vi "Update Z Cursors.vi"(8 "error in (no error)":errorcluster, 11 "Analysis Graph in":refnum<class "Analysis Graph.lvclass">) -> (0 "error out":errorcluster, 3 "Analysis Graph out":refnum<class "Analysis Graph.lvclass">)   [LabVIEW 2023, in "Analysis Graph.lvclass"]
uses:
  Analysis Graph.lvclass
  D:/git/Graph-Classes/source/Series Graph/Series Graph.lvclass
  Series Graph/Series Graph.lvclass/Series Graph.ctl
  Analysis Graph.lvclass/Analysis Graph.ctl
  Series Graph/Series Graph.lvclass
  D:/git/Graph-Classes/source/Detail Graph/Detail Graph.lvclass
  D:/git/Graph-Classes/source/Base Graph/Base Graph.lvclass
  D:/git/Graph-Classes/source/Analysis Graph/Analysis Graph.lvclass
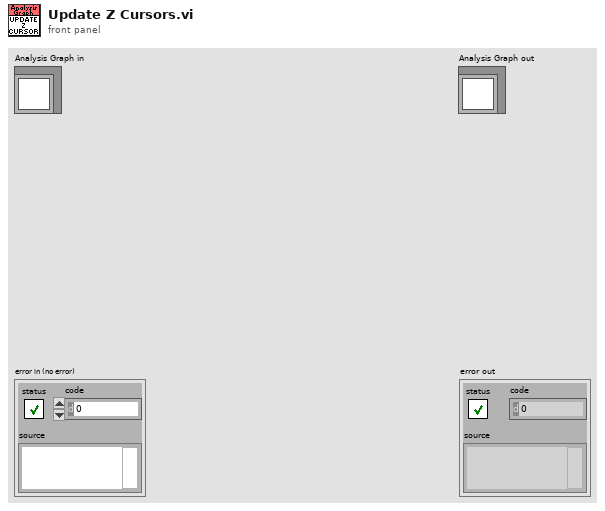
[diagram p1: front panel]
types:
  T1 = cluster{"ROI X":cluster{"Index":u32, "Length":u32}, "ROI Y":cluster{"Index":u32, "Length":u32}, "ROI Z":cluster{"Index":u32, "Length":u32}}
  T2 = typedef "LVCursorListTypeDef.ctl" = cluster{"Name":string, "Color":u32, "Style":u8, "Point Style":u8, "Name Visible":bool, "Allow Drag":bool, "Cursor Mode":u32, "Plot":i32, "Index":i32, "Position":cluster{"X":dbl, "Y":dbl}, "X Scale":u32, "Y Scale":u32, "Watch Plots":i32[], "Watch All Plots":bool, "Plot Area":i32, "Label Offset":cluster{"X":dbl, "Y":dbl}}[]
  T3 = cluster{"Name":string, "Color":u32, "Style":u8, "Point Style":u8, "Name Visible":bool, "Allow Drag":bool, "Cursor Mode":u32, "Plot":i32, "Index":i32, "Position":cluster{"X":dbl, "Y":dbl}, "X Scale":u32, "Y Scale":u32, "Watch Plots":i32[], "Watch All Plots":bool, "Plot Area":i32, "Label Offset":cluster{"X":dbl, "Y":dbl}}
  T4 = cluster{"Name":string, "Color":u32, "Style":u8, "Point Style":u8, "Name Visible":bool, "Allow Drag":bool, "Cursor Mode":u32, "Plot":i32, "Index":i32, "Position":cluster{"X":dbl, "Y":dbl}, "X Scale":u32, "Y Scale":u32, "Watch Plots":i32[], "Watch All Plots":bool, "Plot Area":i32, "Label Offset":cluster{"X":dbl, "Y":dbl}}[]
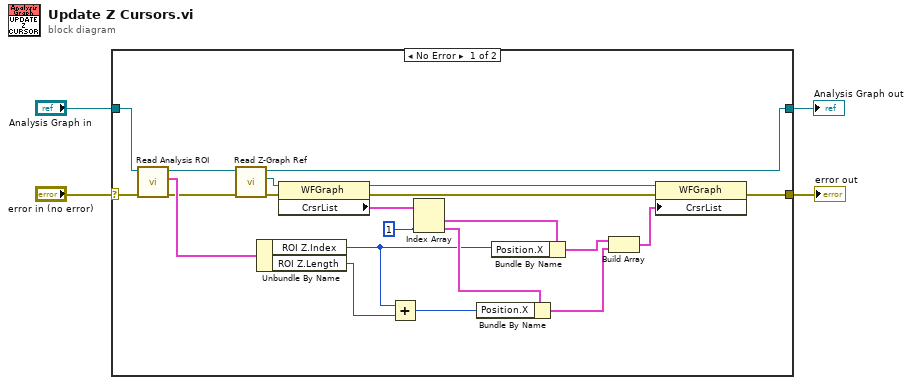
[diagram p0: block diagram]
diagram:
  n1 = case shown="No Error" "error in (no error)" {
    selector: "error in (no error)" -> [w25 w27]
    tunnel: [w11 w27] -> w3
    tunnel: [w7 w26] -> w1
    tunnel: "Analysis Graph in" -> [w8 w26]
    frame No Error {
      n2 = call "Read Analysis ROI.vi"("error in (no error)"=w25, "Analysis Graph in"=w8) -> ("error out"=w5:errorcluster, "ROI XYZ"=w24:T1, "Analysis Graph out"=w6:refnum<class "Analysis Graph.lvclass">)  [unwired: 7 in]
      n3 = call "Read Z-Graph Ref.vi"("error in (no error)"=w5, "Series Graph in"=w6) -> ("error out"=w22:errorcluster, "Z-Graph Ref"=w23:refnum<vi>, "Series Graph out"=w7:refnum<class "Analysis Graph.lvclass">)  [unwired: 7 in]
      n4 = Unbundle By Name(w24) -> ("ROI Z.Index"=w9:u32, "ROI Z.Length"=w17:u32)
      n5 = property class="WFGraph"(reference=w23, error in=w22) -> (reference out=w16:refnum<vi>, error out=w15:errorcluster, "CrsrList"=w21:T2)
      n6 = Add(x=w9, y=w17) -> (x+y=w10:u32)
      n7 = Index Array(array=w21, index #2=1 ("index")) -> (element #1=w19:T3, element #2=w18:T3)  [unwired: 1 in]
      n8 = Bundle By Name(cluster=w18, "Position.X"=w10) -> (w13:T3)
      n9 = Bundle By Name(cluster=w19, "Position.X"=w9) -> (w14:T3)
      n10 = Build Array(w14, w13) -> (w12:T4)
      n11 = property class="WFGraph"(reference=w16, error in=w15, "CrsrList"=w12) -> (error out=w11:errorcluster)  [unwired: 1 out]
    }
    frame Error {
    }
  }
  "error out" <- w3
  "Analysis Graph out" <- w1
